vi "StartPoll.vi"(8 "error in (no error)":errorcluster, 10 "Poll":enum32{"All", "Fast", "Medium", "Slow"}(ring), 11 "Ref":T1) -> (0 "error out":errorcluster, 3 "Ref":T1)   [LabVIEW 2019, in "Diagnostics Host Automation API.lvlib"]
uses:
  Diagnostics Host Automation API.lvlib
  Shared/Types/HostAutomation.Ref.ctl
  <vilib>/NI/STM/TCP/TCP Connection Info.ctl
  <vilib>/NI/STM/SubVIs/MetaDataElement.ctl
  Shared/Types/DTC.Codes.ctl
  <vilib>/NI/NIVS Addon Network Comm/Shared/NI VeriStand Addon Network Comm Shared.lvlib
  <vilib>/NI/STM/NI STM.lvlib
  Shared/Diagnostics Addon Shared.lvlib
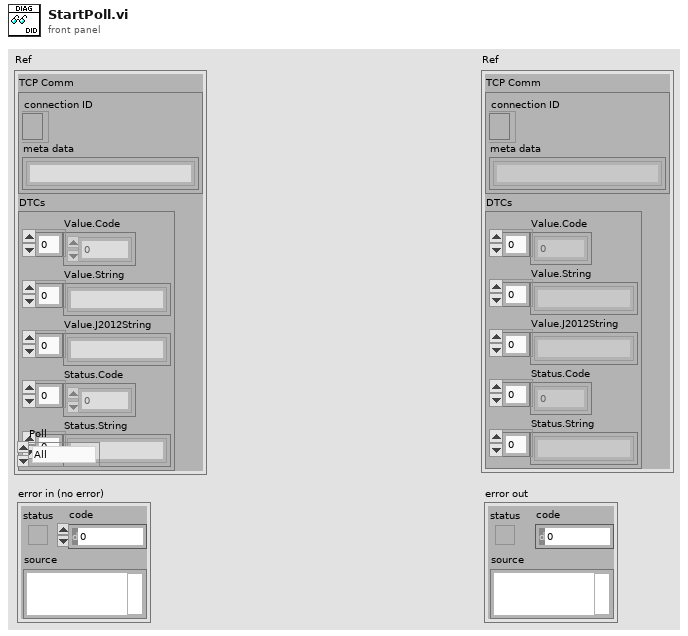
[diagram p1: front panel]
types:
  T1 = typedef "Diagnostics Addon Shared.lvlib/HostAutomation.Ref.ctl" = cluster{"TCP Comm":T2, "DTCs":T4}
  T2 = typedef "NI STM.lvlib/TCP Connection Info.ctl" = cluster{"connection ID":refnum<k5>, "meta data":T3[]}
  T3 = typedef "NI STM.lvlib/MetaDataElement.ctl" = string
  T4 = typedef "Diagnostics Addon Shared.lvlib/DTC.Codes.ctl" = cluster{"Value.Code":dbl[], "Value.String":string[], "Value.J2012String":string[], "Status.Code":dbl[], "Status.String":string[]}
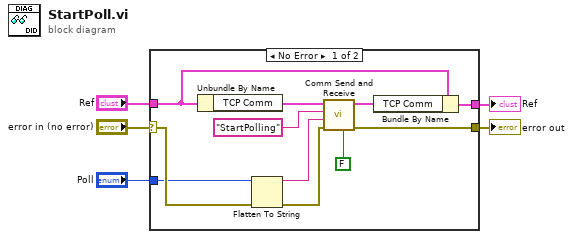
[diagram p0: block diagram]
diagram:
  n1 = case shown="No Error" "error in (no error)" {
    selector: "error in (no error)" -> [w14 w18]
    tunnel: "Ref" -> [w10 w17]
    tunnel: [w8 w17] -> w4
    tunnel: [w7 w18] -> w3
    tunnel: "Poll" -> [w12 _]
    frame No Error {
      n2 = Unbundle By Name(w10) -> ("TCP Comm"=w11:T2)
      n3 = Flatten To String(anything=w12, error in (no error)=w14) -> (data string=w15:string, error out=w13:errorcluster)  [unwired: 2 in, 1 out]
      n4 = call <vilib>:"Comm Send and Receive.vi"("Resp Required?"=FALSE, "error in (no error)"=w13, "Data"=w15, "Name"="StartPolling", "connection info"=w11) -> ("error out"=w7:errorcluster, "connection info"=w9:T2)  [unwired: 3 in, 2 out]
      n5 = Bundle By Name(cluster=w10, "TCP Comm"=w9) -> (w8:T1)
    }
    frame Error {
    }
  }
  "Ref" <- w4
  "error out" <- w3
